vi "Target_Main.vi"() -> ()   [LabVIEW 2021]
uses:
  parametersRT.ctl
panel:
  in  "Parameters":T1={"N_Signals_FIFO"=90, "Input Rate (Hz)"=100.0, "Acq Time (s)"=100000.0, "NumOfWarmupIters"=500, "Size fifo"=500, "Period NCL (ms)"=1000, "Timeout fifo Read"=100, "Size Sent Array"=100}
  out "error out":errorcluster={"status"=TRUE, "code"=56, "source"="UDP Read in Controller_Adrian_Trial.vi->RT_Control_AllIncluded_AngleToPy.vi->Target_Main.vi"}
  # "Before running, zero FB, ESP and Endevco"
  # "Size"
  # "Size Sent Array: The length of data sent in stream for each NCL loop (How many data after every \"Period NCL\")\n      For example, the real-time daq is sampling at 100 Hz (100 data in 1 sec). and Period NCL is 1 sec, \n      then Size Sent Array should be 100 to clean up the RT FIFO. So Input Rate * Period NCL = Size Sent Array"
  # "Timeout fifo Read: timeout for function RT FIFO Read, in ms"
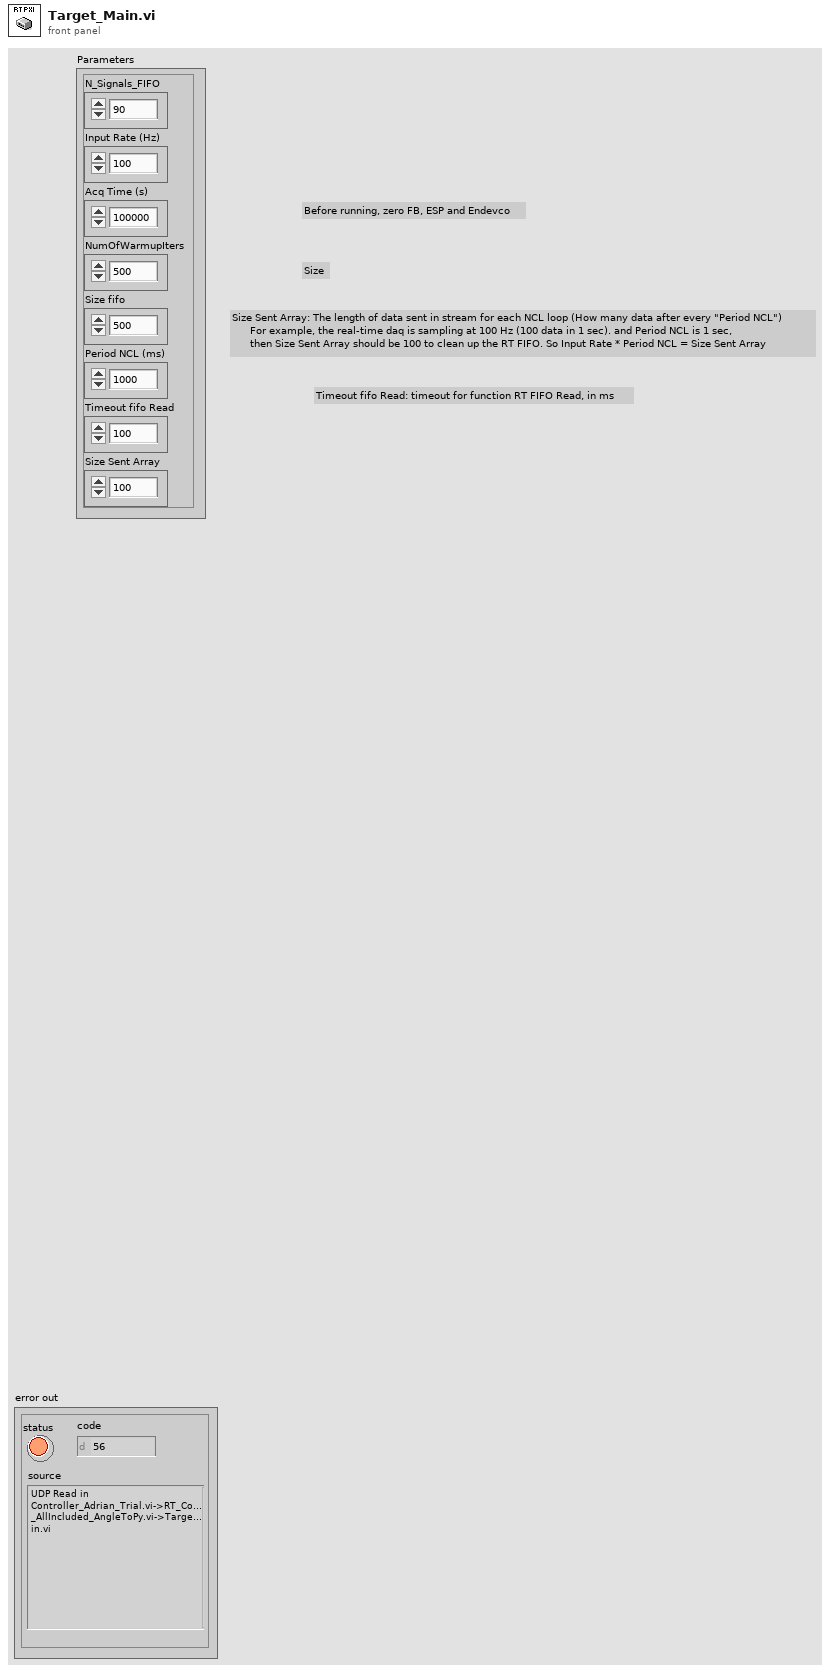
[diagram p1: front panel]
types:
  T1 = typedef "parametersRT.ctl" = cluster{"N_Signals_FIFO":u32, "Input Rate (Hz)":dbl, "Acq Time (s)":dbl, "NumOfWarmupIters":u32, "Size fifo":u32, "Period NCL (ms)":i64, "Timeout fifo Read":i32, "Size Sent Array":i32}
  T2 = cluster{"read mode":enum16{"polling", "blocking"}, "write mode":enum16{"polling", "blocking"}}
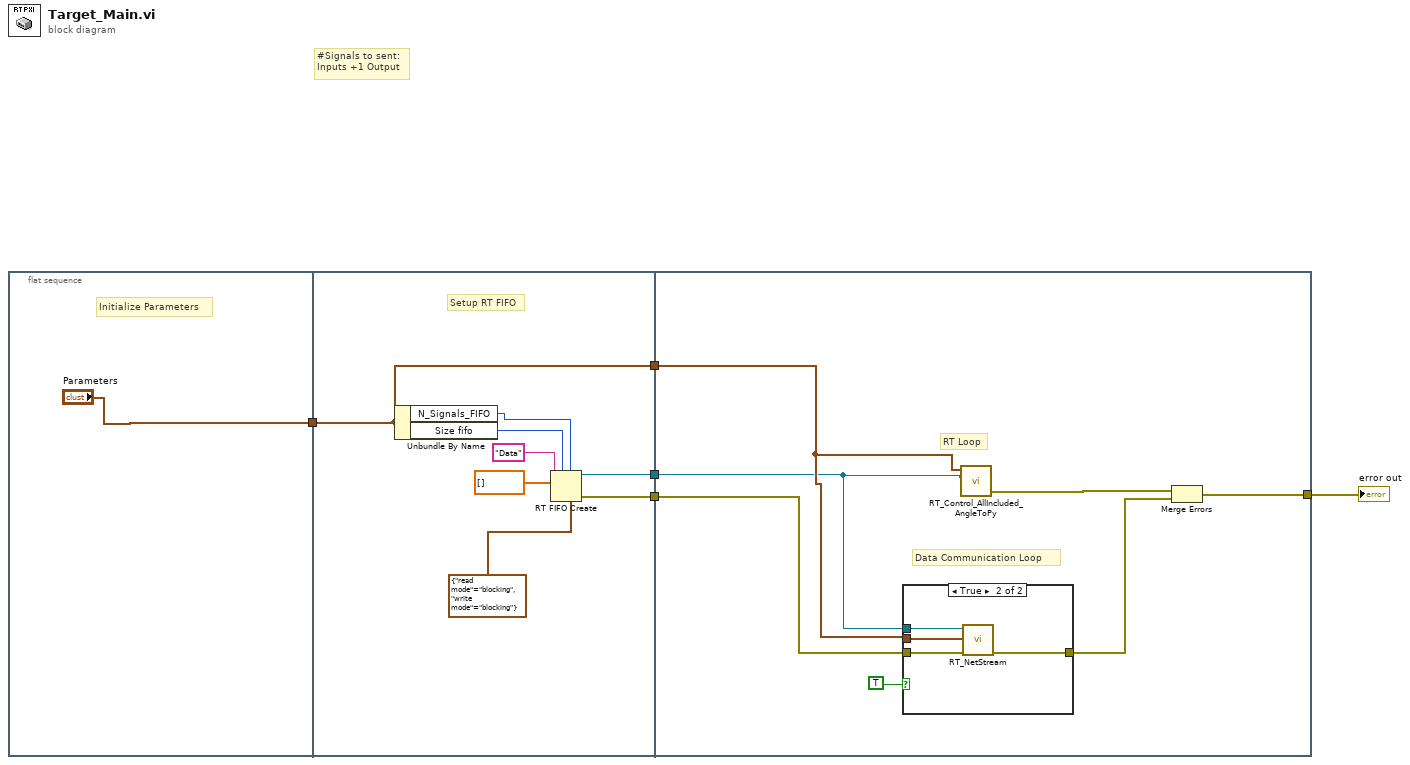
[diagram p0: block diagram]
diagram:
  # "#Signals to sent:\nInputs +1 Output"
  n1 = flat-sequence {
    tunnel: ["Parameters"] -> w1
    tunnel: [w8] -> w5
    tunnel: [w10] -> w4
    tunnel: [w9] -> w3
    tunnel: w1 -> [w8]
    tunnel: w5 -> [w16]
    tunnel: w4 -> [w18]
    tunnel: w3 -> [w15]
    tunnel: [w19] -> w2
    frame #0 {
      # "Initialize Parameters"
    }
    frame #1 {
      # "Setup RT FIFO"
      n2 = Unbundle By Name(w8) -> ("N_Signals_FIFO"=w11:u32, "Size fifo"=w12:u32)
      n3 = RT FIFO Create(0:"Data" ("name (unnamed)"), 1:dbl[] [] ("output array"), 4:w12, 6:w11, 7:T2 {"read mode"=enum."blocking", "write mode"=enum."blocking"} ("r/w modes (polling,polling)")) -> (8:w9:refnum<k33>, 11:w10:errorcluster)  [unwired: 3 in, 1 out]
    }
    frame #2 {
      # "Data Communication Loop"
      # "RT Loop"
      n4 = case shown="True" TRUE ("NTCL") {
        tunnel: [w22 w24] -> w20
        tunnel: w18 -> [w22 w26]
        tunnel: w15 -> [_ w25]
        tunnel: w16 -> [_ w23]
        frame False {
        }
        frame True {
          n5 = call "RT_NetStream.vi"("error in (no error)"=w26, "Parameters"=w23, "rt fifo"=w25) -> ("error out"=w24:errorcluster)  [unwired: 8 in]
        }
      }
      n6 = call "RT_Control_AllIncluded_AngleToPy.vi"("rt fifo"=w15, "Parameters"=w16) -> ("error out"=w17:errorcluster)  [unwired: 8 in, 1 out]
      n7 = Merge Errors(w17, w20) -> (w19:errorcluster)
    }
  }
  "error out" <- w2
